vi "dsdll_status.vi"(8 "error in":errorcluster, 11 "dsdll instance in":T1={"dsdll path"=path "E:/LVprog/DirectSoundDLL/dsdll.dll", "dsdll handle"=[], "output devices"=[], "capture devices"=[]}) -> (0 "error out":errorcluster, 1 "output buffer ok":bool, 2 "output device ok":bool, 3 "dsdll instance out":T1, 4 "input capture ok":bool, 5 "invalid instance handle":bool)   [LabVIEW 2013, in "dsdll.lvlib"]
doc: "Call to get status of DSDLL instance handle. It returns status of output device, output buffer and capture device.\nThis VI can be called from a different thread/process. The 'dsdll instance out' is optional because the function changes nothing in the DSDLL instance."
uses:
  dsdll.lvlib
  dsdll_instance.ctl
  dsdll_device_record.ctl
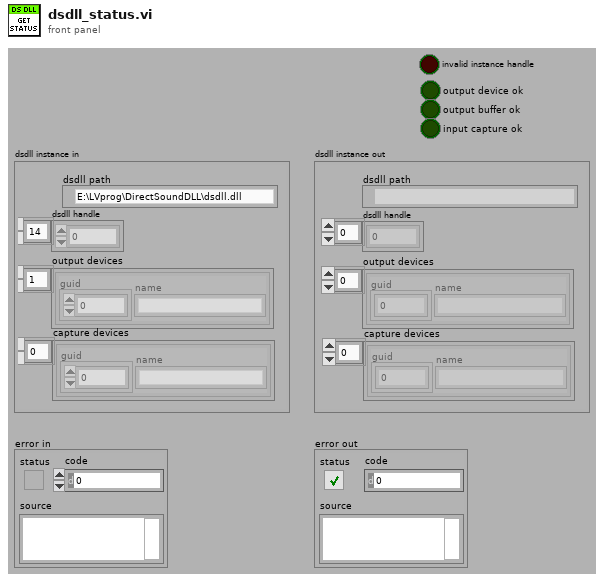
[diagram p1: front panel]
types:
  T1 = typedef "dsdll.lvlib/dsdll_instance.ctl" = cluster{"dsdll path":path, "dsdll handle":u8[], "output devices":T2[], "capture devices":T2[]}
  T2 = typedef "dsdll.lvlib/dsdll_device_record.ctl" = cluster{"guid":u8[], "name":string}
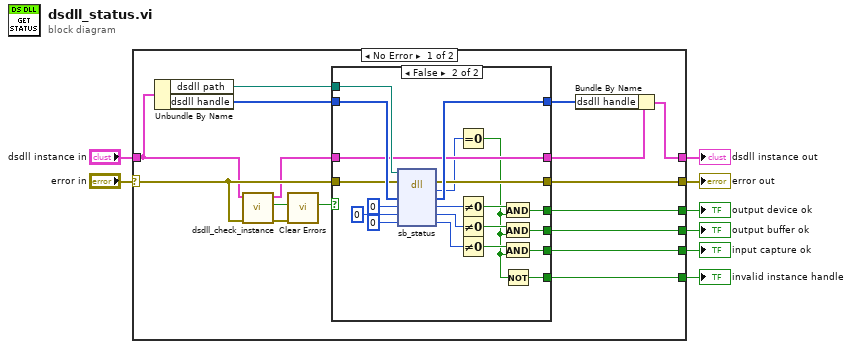
[diagram p0: block diagram]
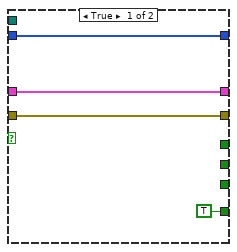
[diagram p2: hidden frame]
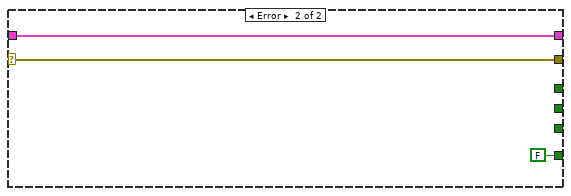
[diagram p3: hidden frame]
diagram:
  n1 = case shown="No Error" "error in" {
    selector: "error in" -> [w13 w50]
    tunnel: "dsdll instance in" -> [w12 w51]
    tunnel: [w22 w50] -> w7
    tunnel: [w19 w51] -> w8
    tunnel: [w18 _] -> w4
    tunnel: [w17 _] -> w3
    tunnel: [w16 _] -> w2
    tunnel: [w14 FALSE] -> w1
    frame No Error {
      n2 = Unbundle By Name(w12) -> ("dsdll path"=w23:path, "dsdll handle"=w15:u8[])
      n3 = call "dsdll_check_instance.vi"("error in"=w13, "dsdll instance in"=w12) -> ("error out"=w9:errorcluster, "empty instance handle"=w10:bool, "dsdll instance out"=w11:T1)  [unwired: 7 in]
      n4 = call <vilib>:"Clear Errors.vi"("error in (no error)"=w9) -> ()  [unwired: 6 in, 1 out]
      n5 = case shown="False" w10 {
        tunnel: w11 -> [w26 w36]
        tunnel: w23 -> [_ w48]
        tunnel: w15 -> [w25 w47]
        tunnel: [w27 w37] -> w22
        tunnel: [w26 w36] -> w21
        tunnel: [w25 w46] -> w20
        tunnel: w13 -> [w27 w45]
        tunnel: [_ w35] -> w18
        tunnel: [_ w34] -> w17
        tunnel: [_ w32] -> w16
        tunnel: [TRUE w28] -> w14
        frame True {
        }
        frame False {
          n6 = dll-call lib="dsdll.dll" fn="sb_status" ("sb_get_handle_size()")(path in=w48, error in=w45, "handle"=w47, "out"=0 ("status"), "out_buffer"=0 ("smpl_pos"), "input"=0 ("smpl_count")) -> (error out=w37:errorcluster, "error"=w30:i32, "handle"=w46:u8[], "out"=w41:i32, "out_buffer"=w39:i32, "input"=w38:i32)  [unwired: 1 in, 1 out]
          n7 = Equal To 0?(x=w30) -> (x = 0?=w29:bool)
          n8 = Not Equal To 0?(x=w41) -> (x != 0?=w40:bool)
          n9 = Not Equal To 0?(x=w39) -> (x != 0?=w33:bool)
          n10 = Not Equal To 0?(x=w38) -> (x != 0?=w31:bool)
          n11 = And(x=w40, y=w29) -> (x .and. y?=w35:bool)
          n12 = And(x=w33, y=w29) -> (x .and. y?=w34:bool)
          n13 = And(x=w31, y=w29) -> (x .and. y?=w32:bool)
          n14 = Not(x=w29) -> (.not. x?=w28:bool)
        }
      }
      n15 = Bundle By Name(cluster=w21, "dsdll handle"=w20) -> (w19:T1)
    }
    frame Error {
    }
  }
  "error out" <- w7
  "dsdll instance out" <- w8
  "output device ok" <- w4
  "output buffer ok" <- w3
  "input capture ok" <- w2
  "invalid instance handle" <- w1
